vi "2 angle_difference_sign.vi"(1 "Angle 2":dbl, 2 "Angle 1":dbl) -> (0 "Difference":dbl)   [LabVIEW 2011]
doc: "Returns the angle between to headings, accounting for wraparound (0 and 355 are 5 degrees apart)"
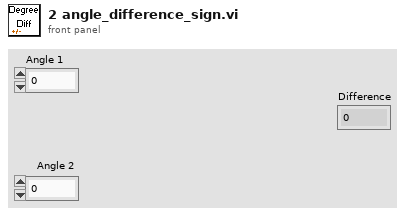
[diagram p1: front panel]
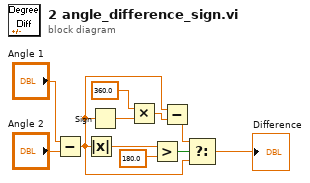
[diagram p0: block diagram]
diagram:
  n1 = Subtract(x="Angle 1", y="Angle 2") -> (x-y=w2:dbl)
  n2 = Absolute Value(x=w2) -> (abs(x)=w8:dbl)
  n3 = Sign(1:w2) -> (0:w5:dbl)
  n4 = Multiply(x=360.0 ("y"), y=w5) -> (x*y=w1:dbl)
  n5 = Greater?(x=w8, y=180.0) -> (0:w9:bool)
  n6 = Subtract(x=w2, y=w1) -> (x-y=w3:dbl)
  n7 = Select(t=w3, s=w9, f=w2) -> (s? t:f=→"Difference":dbl)
